vi "HSBStayInState.vi"(7 "lastCmd":T1) -> (8 "newHSBCmd":T1)   [LabVIEW 2014]
uses:
  Controls/heinzingerSelect.ctl
  <vilib>/rvi/Emulation/niFpgaGetClockAttributes.vi
  <vilib>/rvi/Emulation/niFpgaSctlEmulationGetInTimedLoop.vi
  <vilib>/rvi/Emulation/niFpgaEmulationReportErrorSimple.vi
  heinzingerControlGlobals.vi
  <vilib>/rvi/Emulation/niFpgaCriticalErrorInLSC.vi
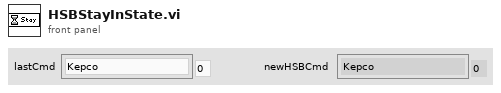
[diagram p1: front panel]
types:
  T1 = typedef "heinzingerSelect.ctl" = enum8{"Kepco", "Heinzinger0", "Heinzinger1", "Heinzinger2", "loading"}
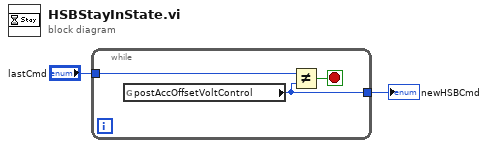
[diagram p0: block diagram]
diagram:
  n1 = while {
    tunnel: "lastCmd" -> [w4]
    tunnel: [w3] -> w1
    stop <- w5 stop-if-true
    n2 = global read "heinzingerControlGlobals.vi" "postAccOffsetVoltControl"() -> (w3:T1)
    n3 = Not Equal?(x=w4, y=w3) -> (x != y?=w5:bool)
  }
  "newHSBCmd" <- w1
